vi "test-Diff-Drive-Accel-Limiter-Test2.vi"(8 "error in (no error)":errorcluster) -> (0 "error out":errorcluster, 3 "All tests passed":bool)   [LabVIEW 2019]
uses:
  <vilib>/Rock Robotics/WPI/ThirdParty/JAS_Junk/TrajLib/MatBuilder_Create.vi
  <vilib>/Rock Robotics/WPI/ThirdParty/JAS_Junk/TrajLib/LinearSystem_New.vi
  <vilib>/Rock Robotics/WPI/ThirdParty/JAS_Junk/TrajLib/MatrixHelper_Zero.vi
  <vilib>/Rock Robotics/WPI/ThirdParty/JAS_Junk/TrajLib/Discretization_DiscretizeAB.vi
  <vilib>/Rock Robotics/WPI/ThirdParty/JAS_Junk/TrajLib/MatrixHelper_CoerceSize.vi
  <vilib>/Rock Robotics/WPI/ThirdParty/JAS_Junk/TrajLib/Matrix_Exp.vi
  <vilib>/Rock Robotics/WPI/ThirdParty/JAS_Junk/TrajLib/Matrix_AssignBlock.vi
  <vilib>/Rock Robotics/WPI/ThirdParty/JAS_Junk/TrajLib/Matrix_ExtractFrom.vi
  <vilib>/Analysis/7linalg.llb/Matrix Exp.vi
  <vilib>/Analysis/7linalg.llb/Real Matrix Exp.vi
  <vilib>/Analysis/Matrix/Numeric/Multiply/Multiply.vi
  <vilib>/Analysis/Matrix/Numeric/Multiply/Multiply - RM,R.vi
  <vilib>/Rock Robotics/WPI/ThirdParty/JAS_Junk/TrajLib/Trajectory_Library.lvlib
panel:
  out "Test 1":bool
  out "Test 2":bool
  out "Test 3":bool
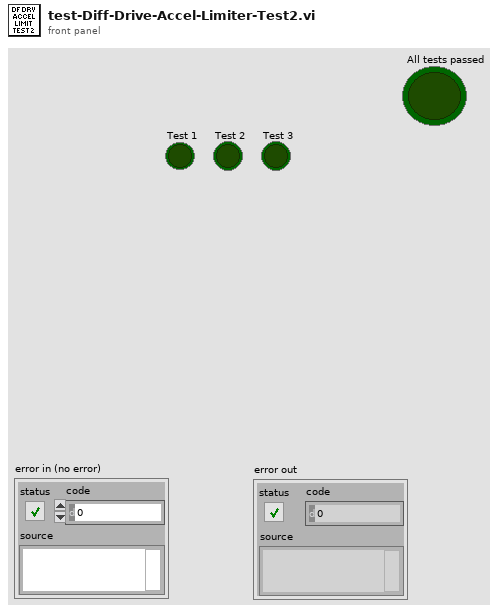
[diagram p1: front panel]
types:
  T1 = typedef "NI_Matrix.lvlib/RealMatrix.ctl" = dbl[][]
  T2 = typedef "Trajectory_Library.lvlib/LINEAR_SYSTEM.ctl" = cluster{"m_A":T1, "m_B":T1, "m_C":T1, "m_D":T1, "States":i32, "Inputs":i32, "Outputs":i32}
  T3 = typedef "Trajectory_Library.lvlib/DIFF_DRIVE_ACCEL_LIMIT.ctl" = cluster{"m_system":T2, "m_trackwidth":dbl, "m_maxLinearAccel":dbl, "m_maxAngularAccel":dbl}
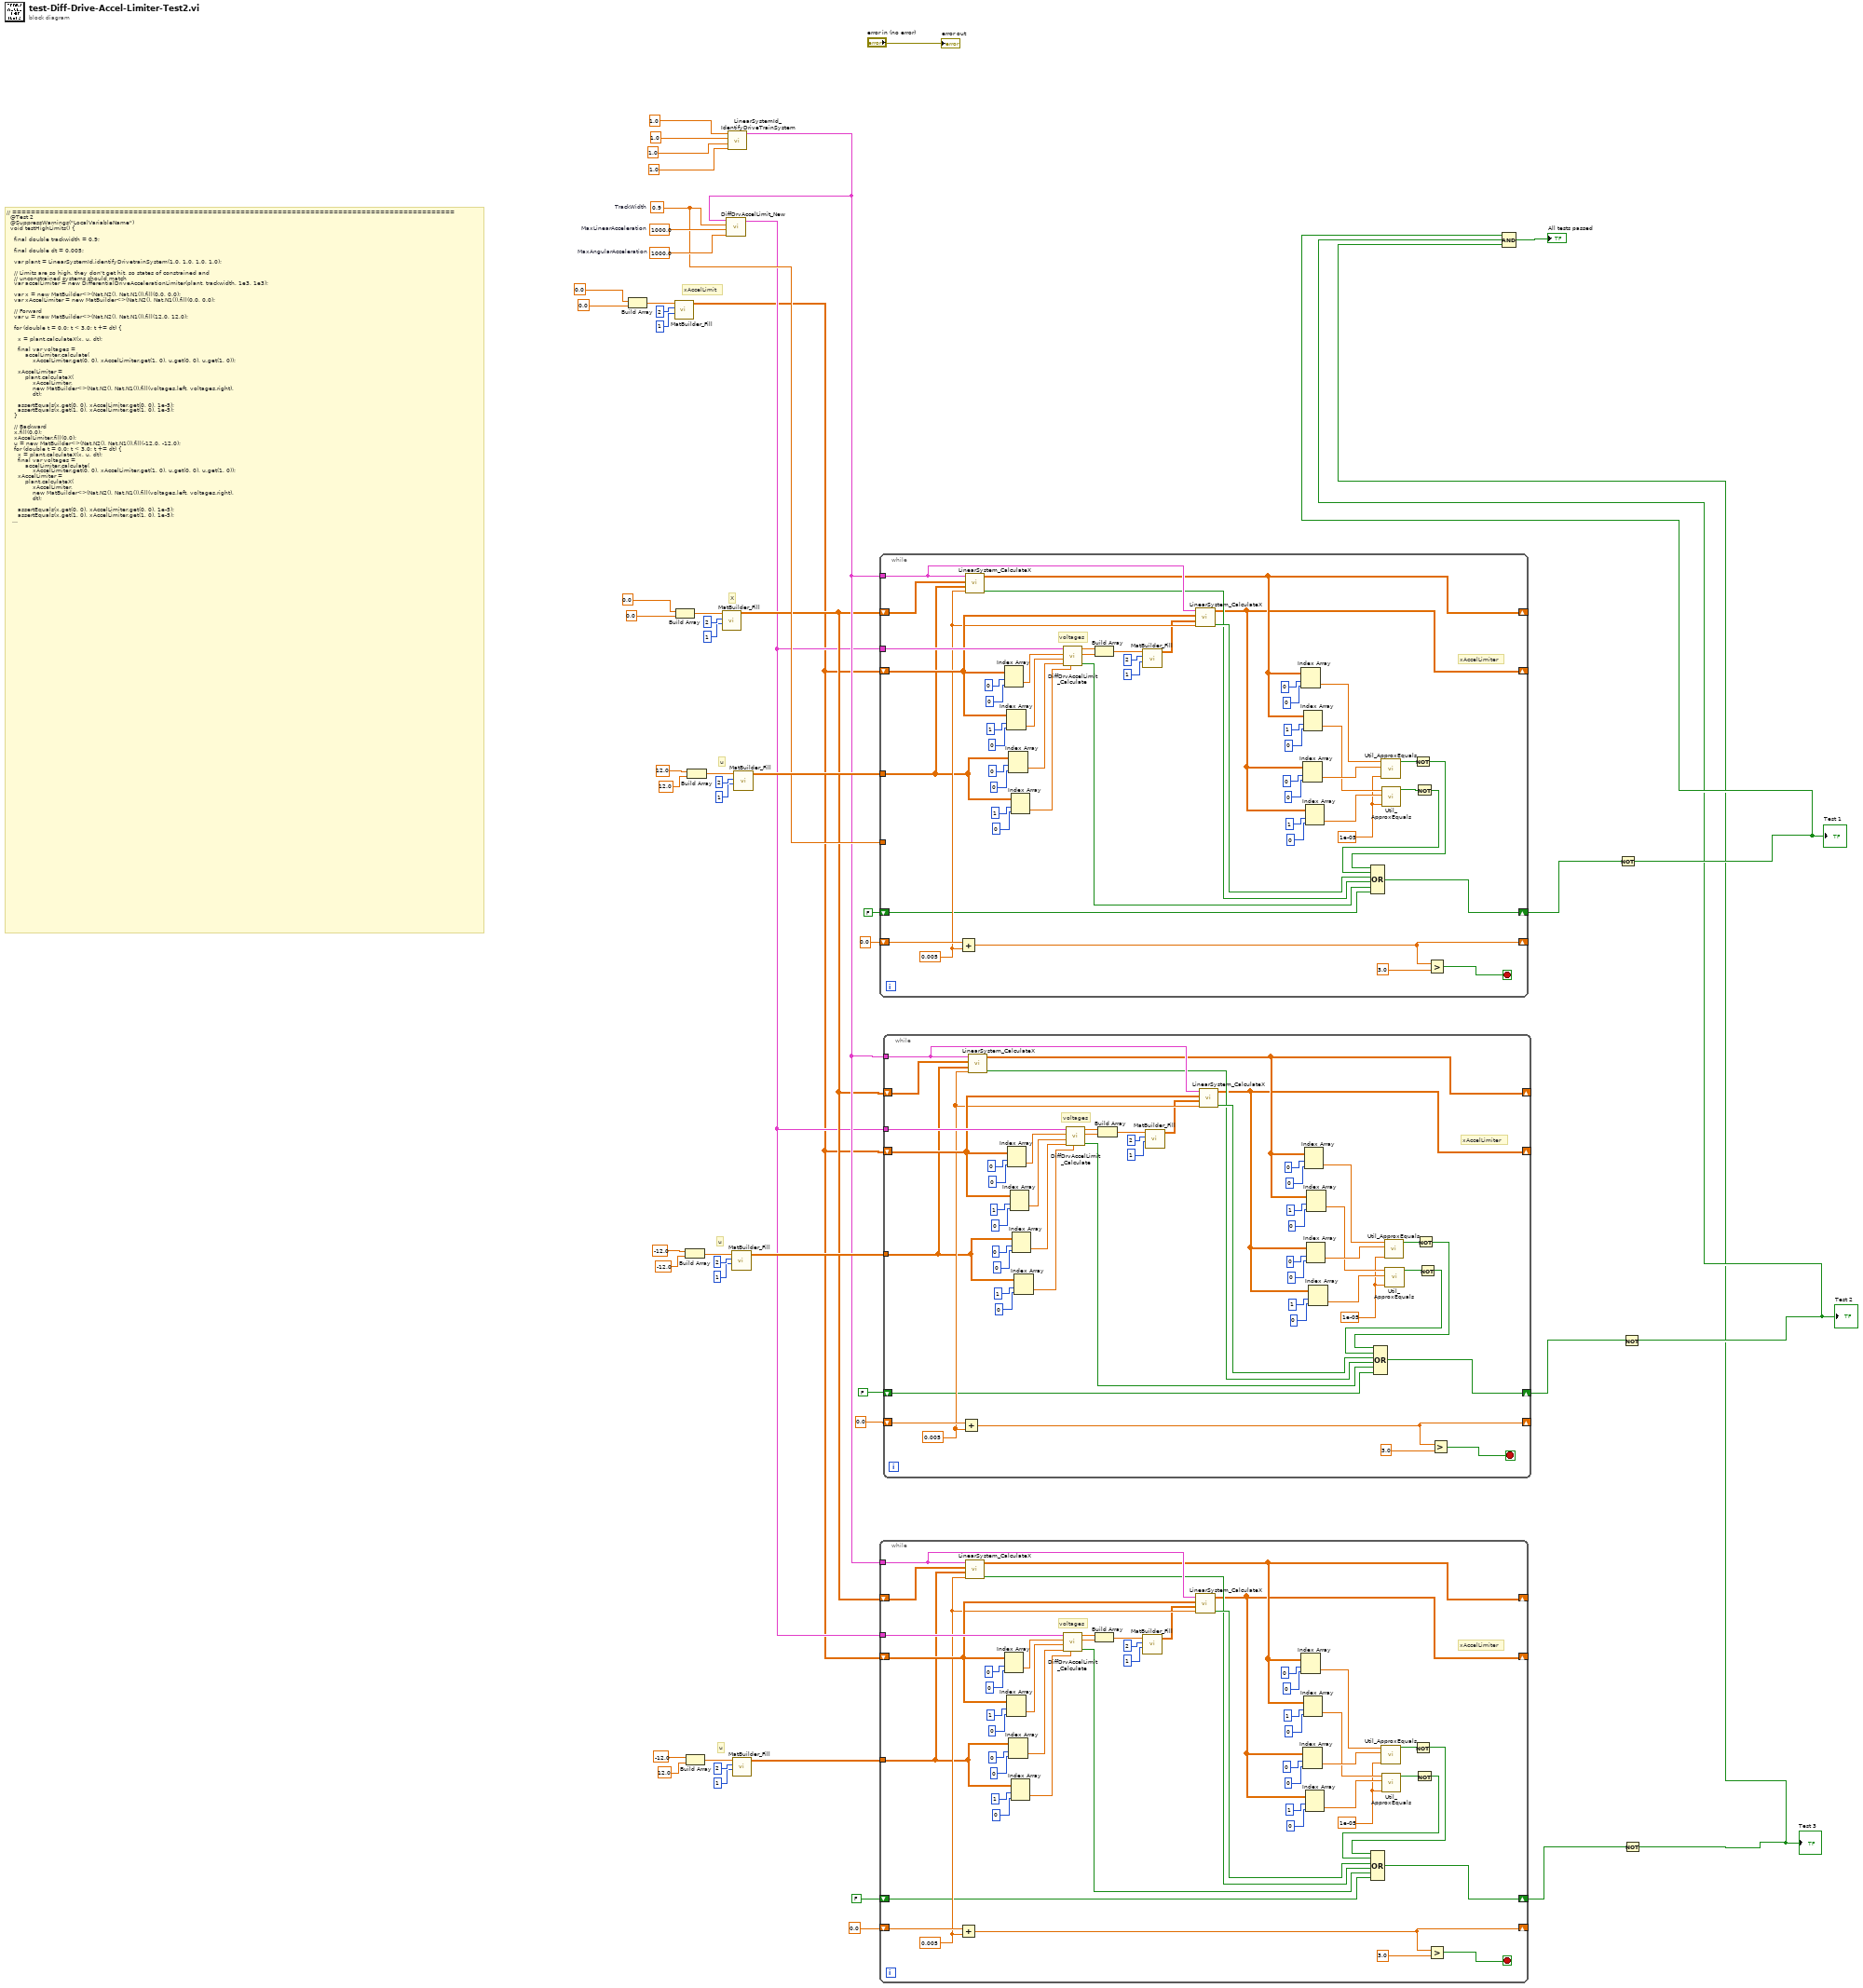
[diagram p0: block diagram]
diagram:
  w17 = 0.9  # TrackWidth
  w18 = 1000.0  # MaxLinearAcceleration
  w19 = 1000.0  # MaxAngularAcceleration
  # "// ===============================================================================================\n  @Test 2\n  @SuppressWarnings(\"LocalVariableName\")\n  void testHighLimits() {\n\n    final double trackwidth = 0.9;\n\n    final double dt = 0.005;\n\n    var plant = LinearSystemId.identifyDrivetrainSystem(1.0, 1.0, 1.0, 1.0);\n\n    // Limits are so high, they don't get hit, so states of constrained and\n    // unconstrained systems should match\n    var accelLimiter = new DifferentialDriveAccelerationLimiter(plant, trackwidth, 1e3, 1e3);\n\n    var x = new MatBuilder<>(Nat.N2(), Nat.N1()).fill(0.0, 0.0);\n    var xAccelLimiter = new MatBuilder<>(Nat.N2(), Nat.N1()).fill(0.0, 0.0);\n\n    // Forward\n    var u = new MatBuilder<>(Nat.N2(), Nat.N1()).fill(12.0, 12.0);\n\n    for (double t = 0.0; t < 3.0; t += dt) {\n\n      x = plant.calculateX(x, u, dt);\n\n      final var voltages =\n          accelLimiter.calculate(\n              xAccelLimiter.get(0, 0), xAccelLimiter.get(1, 0), u.get(0, 0), u.get(1, 0));\n\n      xAccelLimiter =\n          plant.calculateX(\n              xAccelLimiter,\n              new MatBuilder<>(Nat.N2(), Nat.N1()).fill(voltages.left, voltages.right),\n              dt);\n\n      assertEquals(x.get(0, 0), xAccelLimiter.get(0, 0), 1e-5);\n      assertEquals(x.get(1, 0), xAccelLimiter.get(1, 0), 1e-5);\n    }\n\n    // Backward\n    x.fill(0.0);\n    xAccelLimiter.fill(0.0);\n    u = new MatBuilder<>(Nat.N2(), Nat.N1()).fill(-12.0, -12.0);\n    for (double t = 0.0; t < 3.0; t += dt) {\n      x = plant.calculateX(x, u, dt);\n      final var voltages =\n          accelLimiter.calculate(\n              xAccelLimiter.get(0, 0), xAccelLimiter.get(1, 0), u.get(0, 0), u.get(1, 0));\n      xAccelLimiter =\n          plant.calculateX(\n              xAccelLimiter,\n              new MatBuilder<>(Nat.N2(), Nat.N1()).fill(voltages.left, voltages.right),\n              dt);\n\n      assertEquals(x.get(0, 0), xAccelLimiter.get(0, 0), 1e-5);\n      assertEquals(x.get(1, 0), xAccelLimiter.get(1, 0), 1e-5);\n    }\n\n    // Rotate CCW\n    x.fill(0.0);\n    xAccelLimiter.fill(0.0);\n    u = new MatBuilder<>(Nat.N2(), Nat.N1()).fill(-12.0, 12.0);\n    for (double t = 0.0; t < 3.0; t += dt) {\n      x = plant.calculateX(x, u, dt);\n      final var voltages =\n          accelLimiter.calculate(\n              xAccelLimiter.get(0, 0), xAccelLimiter.get(1, 0), u.get(0, 0), u.get(1, 0));\n      xAccelLimiter =\n          plant.calculateX(\n              xAccelLimiter,\n              new MatBuilder<>(Nat.N2(), Nat.N1()).fill(voltages.left, voltages.right),\n              dt);\n\n      assertEquals(x.get(0, 0), xAccelLimiter.get(0, 0), 1e-5);\n      assertEquals(x.get(1, 0), xAccelLimiter.get(1, 0), 1e-5);\n    }\n  }\n}"
  # "u"
  # "u"
  # "u"
  # "xAccelLimit"
  # "X"
  n1 = Build Array(0.0 ("element"), 0.0 ("element")) -> (w43:dbl[])
  n2 = call <vilib>:"MatBuilder_Fill.vi"("Columns"=1, "Rows"=2, "Value List"=w43) -> ("output matrix"=w6:T1)  [unwired: 8 in]
  n3 = Build Array(0.0 ("element"), 0.0 ("element")) -> (w48:dbl[])
  n4 = Build Array(-12.0 ("element"), -12.0 ("element")) -> (w29:dbl[])
  n5 = Build Array(-12.0 ("element"), 12.0 ("element")) -> (w24:dbl[])
  n6 = Build Array(12.0 ("element"), 12.0 ("element")) -> (w38:dbl[])
  n7 = call <vilib>:"MatBuilder_Fill.vi"("Columns"=1, "Rows"=2, "Value List"=w48) -> ("output matrix"=w8:T1)  [unwired: 8 in]
  n8 = call <vilib>:"LinearSystemId_IdentifyDriveTrainSystem.vi"("kAAngular"=1.0 ("rbMeters"), "kVAngular"=1.0 ("rMeters"), "kALinear"=1.0 ("MassKg"), "kVLinear"=1.0 ("JKgMetersSquared")) -> ("Linearsystem"=w9:T2)  [unwired: 6 in, 1 out]
  n9 = call <vilib>:"DiffDrvAccelLimit_New.vi"("MaxAngularAcceleration"=w19, "MaxLinearAcceleration"=w18, "TrackWidth"=w17, "LINEARSYSTEM"=w9) -> ("outDiffDriveAccelLimit"=w7:T3)  [unwired: 7 in]
  n10 = call <vilib>:"MatBuilder_Fill.vi"("Columns"=1, "Rows"=2, "Value List"=w29) -> ("output matrix"=w11:T1)  [unwired: 8 in]
  n11 = call <vilib>:"MatBuilder_Fill.vi"("Columns"=1, "Rows"=2, "Value List"=w24) -> ("output matrix"=w5:T1)  [unwired: 8 in]
  n12 = call <vilib>:"MatBuilder_Fill.vi"("Columns"=1, "Rows"=2, "Value List"=w38) -> ("output matrix"=w32:T1)  [unwired: 8 in]
  n13 = while {
    shift-right: [w102] -> _
    shift-left: 0.0 -> [w105]
    tunnel: w9 -> [w76]
    tunnel: w32 -> [w74]
    shift-right: [w64] -> _
    shift-left: w8 -> [w101]
    tunnel: w7 -> [w100]
    shift-right: [w63] -> _
    shift-left: w6 -> [w87]
    tunnel: w17 -> [_]
    shift-right: [w69] -> w30
    shift-left: FALSE -> [w70]
    stop <- w104 stop-if-true
    w58 = 1e-05 ("Tolerance")
    w81 = 0.005
    # "voltages"
    # "xAccelLimiter"
    n14 = Add(x=w105, y=w81) -> (x+y=w102:dbl)
    n15 = call <vilib>:"LinearSystem_CalculateX.vi"("dT_Seconds"=w81, "ClampedU"=w74, "X"=w101, "Linearsystem"=w76) -> ("Error"=w72:bool, "outX"=w64:T1)  [unwired: 6 in]
    n16 = Index Array(array=w87, index (row)=0, index (col)=0) -> (element=w95:dbl)
    n17 = Index Array(array=w87, index (row)=1, index (col)=0) -> (element=w94:dbl)
    n18 = Index Array(array=w74, index (row)=0, index (col)=0) -> (element=w89:dbl)
    n19 = Index Array(array=w74, index (row)=1, index (col)=0) -> (element=w88:dbl)
    n20 = call <vilib>:"DiffDrvAccelLimit_Calculate.vi"("RightVoltage"=w88, "LeftVoltage"=w89, "RightVelocity"=w94, "LeftVelocity"=w95, "inDiffDriveAccelLimit"=w100) -> ("Error"=w71:bool, "NewRightVoltage"=w82:dbl, "NewLeftVoltage"=w83:dbl)  [unwired: 4 in]
    n21 = Build Array(w83, w82) -> (w86:dbl[])
    n22 = call <vilib>:"MatBuilder_Fill.vi"("Columns"=1, "Rows"=2, "Value List"=w86) -> ("output matrix"=w75:T1)  [unwired: 8 in]
    n23 = call <vilib>:"LinearSystem_CalculateX.vi"("dT_Seconds"=w81, "ClampedU"=w75, "X"=w87, "Linearsystem"=w76) -> ("Error"=w73:bool, "outX"=w63:T1)  [unwired: 6 in]
    n24 = Index Array(array=w64, index (row)=0, index (col)=0) -> (element=w62:dbl)
    n25 = Index Array(array=w63, index (row)=0, index (col)=0) -> (element=w61:dbl)
    n26 = Index Array(array=w64, index (row)=1, index (col)=0) -> (element=w60:dbl)
    n27 = Index Array(array=w63, index (row)=1, index (col)=0) -> (element=w59:dbl)
    n28 = call <vilib>:"Util_ApproxEquals.vi"("Tolerance"=w58, "Value 2"=w61, "Value 1"=w62) -> ("ApproxEquals"=w56:bool)  [unwired: 8 in]
    n29 = call <vilib>:"Util_ApproxEquals.vi"("Tolerance"=w58, "Value 2"=w59, "Value 1"=w60) -> ("ApproxEquals"=w57:bool)  [unwired: 8 in]
    n30 = Not(x=w56) -> (.not. x?=w54:bool)
    n31 = Not(x=w57) -> (.not. x?=w55:bool)
    n32 = Compound Arithmetic op=OR(w54, w55, w73, w72, w71, w70) -> (w69:bool)
    n33 = Greater?(x=w102, y=3.0) -> (0:w104:bool)
  }
  n34 = while {
    shift-right: [w154] -> _
    shift-left: 0.0 -> [w157]
    tunnel: w9 -> [w128]
    tunnel: w5 -> [w126]
    shift-right: [w116] -> _
    shift-left: w8 -> [w153]
    tunnel: w7 -> [w152]
    shift-right: [w115] -> _
    shift-left: w6 -> [w139]
    shift-right: [w121] -> w2
    shift-left: FALSE -> [w122]
    stop <- w156 stop-if-true
    w110 = 1e-05 ("Tolerance")
    w133 = 0.005
    # "voltages"
    # "xAccelLimiter"
    n35 = Add(x=w157, y=w133) -> (x+y=w154:dbl)
    n36 = call <vilib>:"LinearSystem_CalculateX.vi"("dT_Seconds"=w133, "ClampedU"=w126, "X"=w153, "Linearsystem"=w128) -> ("Error"=w124:bool, "outX"=w116:T1)  [unwired: 6 in]
    n37 = Index Array(array=w139, index (row)=0, index (col)=0) -> (element=w147:dbl)
    n38 = Index Array(array=w139, index (row)=1, index (col)=0) -> (element=w146:dbl)
    n39 = Index Array(array=w126, index (row)=0, index (col)=0) -> (element=w141:dbl)
    n40 = Index Array(array=w126, index (row)=1, index (col)=0) -> (element=w140:dbl)
    n41 = call <vilib>:"DiffDrvAccelLimit_Calculate.vi"("RightVoltage"=w140, "LeftVoltage"=w141, "RightVelocity"=w146, "LeftVelocity"=w147, "inDiffDriveAccelLimit"=w152) -> ("Error"=w123:bool, "NewRightVoltage"=w134:dbl, "NewLeftVoltage"=w135:dbl)  [unwired: 4 in]
    n42 = Build Array(w135, w134) -> (w138:dbl[])
    n43 = call <vilib>:"MatBuilder_Fill.vi"("Columns"=1, "Rows"=2, "Value List"=w138) -> ("output matrix"=w127:T1)  [unwired: 8 in]
    n44 = call <vilib>:"LinearSystem_CalculateX.vi"("dT_Seconds"=w133, "ClampedU"=w127, "X"=w139, "Linearsystem"=w128) -> ("Error"=w125:bool, "outX"=w115:T1)  [unwired: 6 in]
    n45 = Index Array(array=w116, index (row)=0, index (col)=0) -> (element=w114:dbl)
    n46 = Index Array(array=w115, index (row)=0, index (col)=0) -> (element=w113:dbl)
    n47 = Index Array(array=w116, index (row)=1, index (col)=0) -> (element=w112:dbl)
    n48 = Index Array(array=w115, index (row)=1, index (col)=0) -> (element=w111:dbl)
    n49 = call <vilib>:"Util_ApproxEquals.vi"("Tolerance"=w110, "Value 2"=w113, "Value 1"=w114) -> ("ApproxEquals"=w108:bool)  [unwired: 8 in]
    n50 = call <vilib>:"Util_ApproxEquals.vi"("Tolerance"=w110, "Value 2"=w111, "Value 1"=w112) -> ("ApproxEquals"=w109:bool)  [unwired: 8 in]
    n51 = Not(x=w108) -> (.not. x?=w106:bool)
    n52 = Not(x=w109) -> (.not. x?=w107:bool)
    n53 = Compound Arithmetic op=OR(w106, w107, w125, w124, w123, w122) -> (w121:bool)
    n54 = Greater?(x=w154, y=3.0) -> (0:w156:bool)
  }
  n55 = while {
    shift-right: [w206] -> _
    shift-left: 0.0 -> [w209]
    tunnel: w9 -> [w180]
    tunnel: w11 -> [w178]
    shift-right: [w168] -> _
    shift-left: w8 -> [w205]
    tunnel: w7 -> [w204]
    shift-right: [w167] -> _
    shift-left: w6 -> [w191]
    shift-right: [w173] -> w14
    shift-left: FALSE -> [w174]
    stop <- w208 stop-if-true
    w162 = 1e-05 ("Tolerance")
    w185 = 0.005
    # "voltages"
    # "xAccelLimiter"
    n56 = Add(x=w209, y=w185) -> (x+y=w206:dbl)
    n57 = call <vilib>:"LinearSystem_CalculateX.vi"("dT_Seconds"=w185, "ClampedU"=w178, "X"=w205, "Linearsystem"=w180) -> ("Error"=w176:bool, "outX"=w168:T1)  [unwired: 6 in]
    n58 = Index Array(array=w191, index (row)=0, index (col)=0) -> (element=w199:dbl)
    n59 = Index Array(array=w191, index (row)=1, index (col)=0) -> (element=w198:dbl)
    n60 = Index Array(array=w178, index (row)=0, index (col)=0) -> (element=w193:dbl)
    n61 = Index Array(array=w178, index (row)=1, index (col)=0) -> (element=w192:dbl)
    n62 = call <vilib>:"DiffDrvAccelLimit_Calculate.vi"("RightVoltage"=w192, "LeftVoltage"=w193, "RightVelocity"=w198, "LeftVelocity"=w199, "inDiffDriveAccelLimit"=w204) -> ("Error"=w175:bool, "NewRightVoltage"=w186:dbl, "NewLeftVoltage"=w187:dbl)  [unwired: 4 in]
    n63 = Build Array(w187, w186) -> (w190:dbl[])
    n64 = call <vilib>:"MatBuilder_Fill.vi"("Columns"=1, "Rows"=2, "Value List"=w190) -> ("output matrix"=w179:T1)  [unwired: 8 in]
    n65 = call <vilib>:"LinearSystem_CalculateX.vi"("dT_Seconds"=w185, "ClampedU"=w179, "X"=w191, "Linearsystem"=w180) -> ("Error"=w177:bool, "outX"=w167:T1)  [unwired: 6 in]
    n66 = Index Array(array=w168, index (row)=0, index (col)=0) -> (element=w166:dbl)
    n67 = Index Array(array=w167, index (row)=0, index (col)=0) -> (element=w165:dbl)
    n68 = Index Array(array=w168, index (row)=1, index (col)=0) -> (element=w164:dbl)
    n69 = Index Array(array=w167, index (row)=1, index (col)=0) -> (element=w163:dbl)
    n70 = call <vilib>:"Util_ApproxEquals.vi"("Tolerance"=w162, "Value 2"=w165, "Value 1"=w166) -> ("ApproxEquals"=w160:bool)  [unwired: 8 in]
    n71 = call <vilib>:"Util_ApproxEquals.vi"("Tolerance"=w162, "Value 2"=w163, "Value 1"=w164) -> ("ApproxEquals"=w161:bool)  [unwired: 8 in]
    n72 = Not(x=w160) -> (.not. x?=w158:bool)
    n73 = Not(x=w161) -> (.not. x?=w159:bool)
    n74 = Compound Arithmetic op=OR(w158, w159, w177, w176, w175, w174) -> (w173:bool)
    n75 = Greater?(x=w206, y=3.0) -> (0:w208:bool)
  }
  n76 = Not(x=w30) -> (.not. x?=w15:bool)
  "Test 1" <- w15
  n77 = Not(x=w14) -> (.not. x?=w10:bool)
  "Test 2" <- w10
  n78 = Not(x=w2) -> (.not. x?=w1:bool)
  "Test 3" <- w1
  n79 = Compound Arithmetic op=AND(w15, w10, w1) -> (→"All tests passed":bool)
  "error out" <- "error in (no error)"
